vi "Spreadsheet Item to String Array.vi"(11 "Spreadsheet Item (ASCII)":string) -> (2 "Strings [] (ASCII)":string[](array[string]))   [LabVIEW 2013, in "SET Project Data.lvlib"]
uses:
  SET Project Data.lvlib
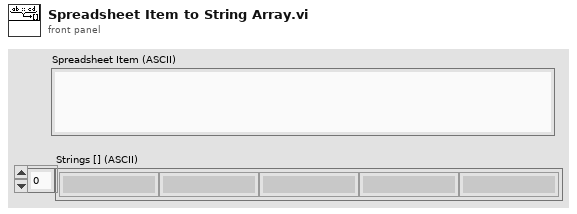
[diagram p1: front panel]
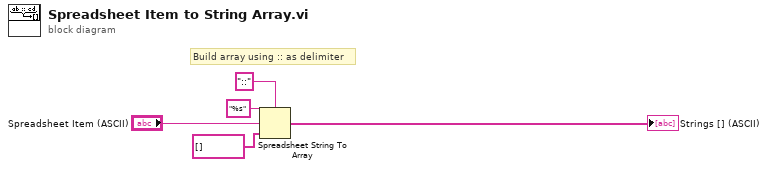
[diagram p0: block diagram]
diagram:
  # "Build array using :: as delimiter"
  n1 = Spreadsheet String To Array(delimiter (Tab)="::", format string="%s", spreadsheet string="Spreadsheet Item (ASCII)", array type (2D Dbl)=string[] []) -> (array=→"Strings [] (ASCII)":string[])
